vi "Get Current Position.vi"(8 "error in (no error)":errorcluster, 11 "FINE SIM Motion Axis":refnum<class "FINE SIM Motion Axis.lvclass">) -> (0 "error out":errorcluster, 2 "Current Position":dbl, 3 "FINE SIM Motion Axis":refnum<class "FINE SIM Motion Axis.lvclass">)   [LabVIEW 2022 SP3, in "FINE SIM Motion Axis.lvclass"]
uses:
  FINE SIM Motion Axis.lvclass
  FINE SIM Motion Axis.lvclass/FINE SIM Motion Axis.ctl
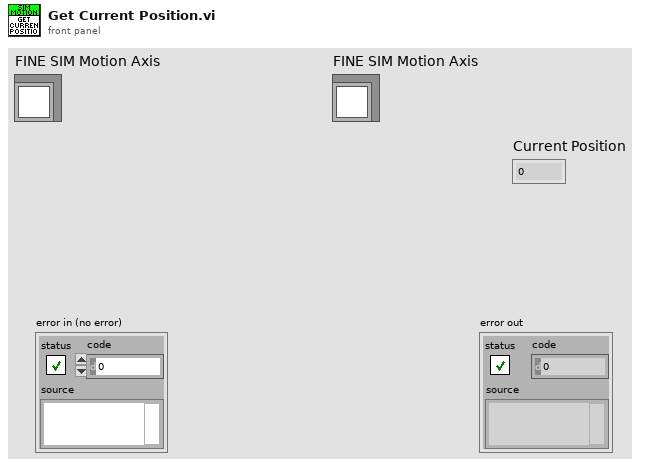
[diagram p1: front panel]
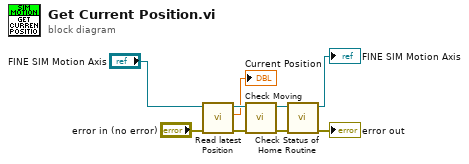
[diagram p0: block diagram]
diagram:
  n1 = call-dynamic "Read latest Position.vi"("error in (no error)"="error in (no error)", "FINE SIM Motion Axis"="FINE SIM Motion Axis") -> ("error out"=w7:errorcluster, "Current Position"=→"Current Position":dbl, "FINE SIM Motion Axis"=w9:refnum<class "FINE SIM Motion Axis.lvclass">)  [unwired: 7 in]
  n2 = call "Check Moving.vi"("error in (no error)"=w7, "FINE SIM Motion Axis"=w9) -> ("error out"=w6:errorcluster, "FINE SIM Motion Axis"=w5:refnum<class "FINE SIM Motion Axis.lvclass">)  [unwired: 8 in]
  n3 = call "Check Status of Home Routine.vi"("error in (no error)"=w6, "FINE SIM Motion Axis"=w5) -> ("error out"=→"error out":errorcluster, "FINE SIM Motion Axis"=→"FINE SIM Motion Axis":refnum<class "FINE SIM Motion Axis.lvclass">)  [unwired: 8 in]
